vi "processResult.vi"(8 "error in":errorcluster, 10 "TestResult in":refnum<class "TestResult.lvclass">, 11 "TextTestRunner in":refnum<class "TextTestRunner.JUnitXML.lvclass">) -> (0 "error out":errorcluster, 2 "TestResult out":refnum<class "TestResult.lvclass">, 3 "TextTestRunner out":refnum<class "TextTestRunner.JUnitXML.lvclass">)   [LabVIEW 2011, in "TextTestRunner.JUnitXML.lvclass"]
uses:
  TextTestRunner.JUnitXML.lvclass
  <vilib>/addons/_JKI Toolkits/VI Tester/TestResult.llb/TestResult.lvclass
  _TextTestResult.Ant/_TextTestResult.JUnitXML.lvclass
  <vilib>/addons/_JKI Toolkits/VI Tester/TextTestRunner.llb/TextTestRunner.lvclass
  TextTestRunner.JUnitXML.lvclass/TextTestRunner.JUnitXML.ctl
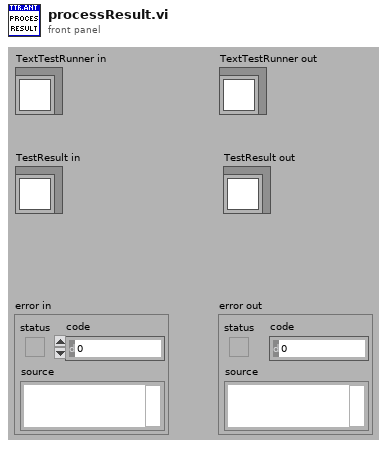
[diagram p1: front panel]
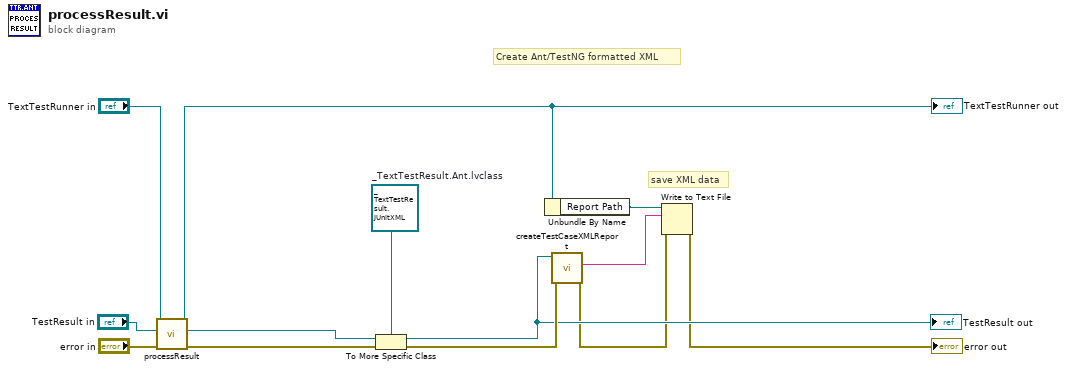
[diagram p0: block diagram]
diagram:
  w13 = refnum<class "_TextTestResult.JUnitXML.lvclass"> refnum  # _TextTestResult.Ant.lvclass
  # "save XML data"
  # "Create Ant/TestNG formatted XML"
  n1 = call-parent "processResult.vi"("error in"="error in", "TestResult in"="TestResult in", "TextTestRunner in"="TextTestRunner in") -> ("error out"=w1:errorcluster, "TestResult out"=w10:refnum<class "TestResult.lvclass">, "TextTestRunner out"=w2:refnum<class "TextTestRunner.JUnitXML.lvclass">)  [unwired: 6 in]
  "TextTestRunner out" <- w2
  n2 = To More Specific Class(target class=w13, reference=w10, error in=w1) -> (specific class reference=w7:refnum<class "_TextTestResult.JUnitXML.lvclass">, error out=w8:errorcluster)
  "TestResult out" <- w7
  n3 = Unbundle By Name(w2) -> ("Report Path"=w6:path)
  n4 = call "createTestCaseXMLReport.vi"("error in (no error)"=w8, "TestTestResult.Ant"=w7) -> ("error out"=w4:errorcluster, "XML Report Data"=w5:string)  [unwired: 8 in]
  n5 = Write to Text File(file (use dialog)=w6, text=w5, error in=w4) -> (error out=→"error out":errorcluster)  [unwired: 1 in, 2 out]
